vi "MPExxx_close.vi"(1 "error in (no error)":errorcluster, 2 "VISA session":refnum<visa-resource-name>) -> (0 "error out":errorcluster)   [LabVIEW 2017]
doc: "This VI closes the I/O interface with the instrument."
panel:
  # "MAGNA-POWER"
  # "Electronics"
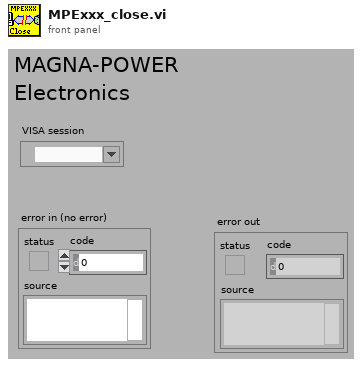
[diagram p1: front panel]
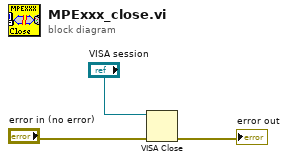
[diagram p0: block diagram]
diagram:
  n1 = VISA Close(VISA resource name="VISA session", error in (no error)="error in (no error)") -> (error out=→"error out":errorcluster)
